vi "Image Difference Global.vi"() -> ()   [LabVIEW 2010, in "Image Difference Custom Device.lvlib"]
uses:
  Image Difference Custom Device.lvlib
panel:
  in  "Subtraction File":string="Subtraction File"
  in  "Channel Type":string="Channel Type"
  in  "ROI Value":string="ROI Value"
  in  "Recent Image":string="Recent Image"
  in  "Camera Path":string="Camera Path"
  in  "Camera Properties":string="Camera Properties"
  in  "Delete Protected GUID":string="7C871B01-1266-4EDB-A195-BFBED06C858B"
  in  "Main Page GUID":string="50F80278-6725-2182-4F44-08B623EAD1F8"
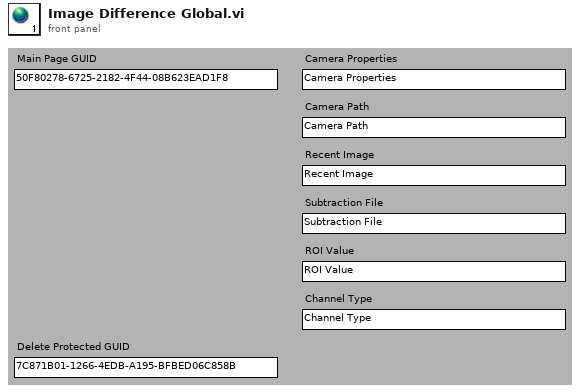
[diagram p1: front panel]
diagram:
